vi "stop.vi"(8 "error in (no error)":errorcluster, 11 "control references in":T1) -> (0 "error out":errorcluster, 3 "control references out":T1)   [LabVIEW 2010]
uses:
  type_definitions/clusters/controls_refs.ctl
  common/classes/GenericToplevelComponent/GenericToplevelComponent/GenericToplevelComponent.lvclass
  type_definitions/enumerations/main_control_types.ctl
  components/ImagingMode/GenericImagingMode/GenericImagingMode/GenericImagingMode.lvclass
  components/ExperimentController/GenericExperimentController/GenericExperimentController/GenericExperimentController.lvclass
  global_variables.vi
  common/classes/GenericComponent/GenericComponent/class_data.vi
  common/classes/GenericComponent/GenericComponent/GenericComponent.lvclass
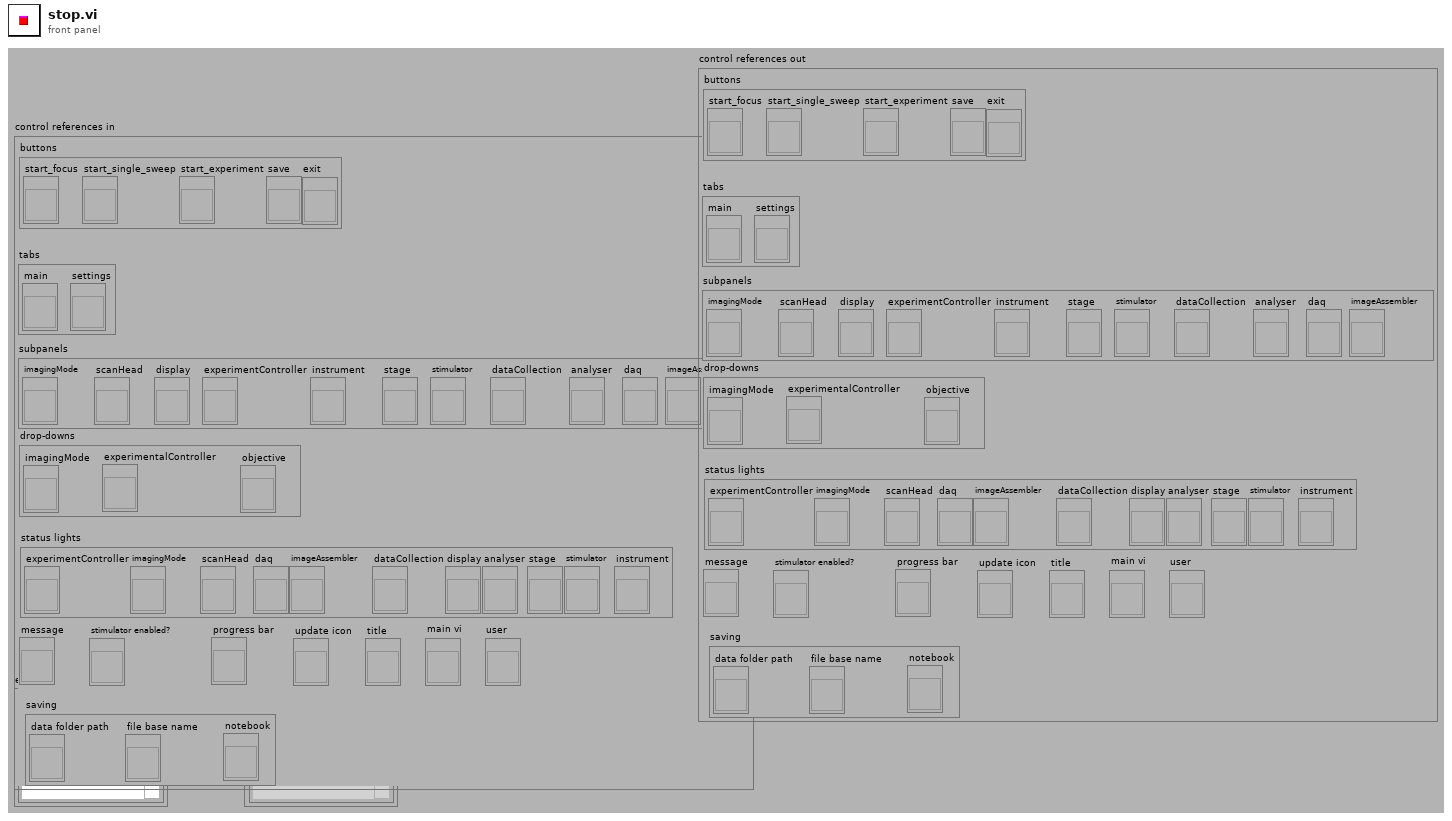
[diagram p1: front panel]
types:
  T1 = typedef "controls_refs.ctl" = cluster{"buttons":cluster{"start_focus":refnum<vi>, "start_single_sweep":refnum<vi>, "start_experiment":refnum<vi>, "save":refnum<vi>, "exit":refnum<vi>}, "tabs":cluster{"main":refnum<vi>, "settings":refnum<vi>}, "subpanels":cluster{"imagingMode":refnum<vi>, "scanHead":refnum<vi>, "display":refnum<vi>, "experimentController":refnum<vi>, "instrument":refnum<vi>, "stage":refnum<vi>, "stimulator":refnum<vi>, "dataCollection":refnum<vi>, "analyser":refnum<vi>, "daq":refnum<vi>, "imageAssembler":refnum<vi>}, "drop-downs":cluster{"imagingMode":refnum<vi>, "experimentalController":refnum<vi>, "objective":refnum<vi>}, "status lights":cluster{"experimentController":refnum<vi>, "imagingMode":refnum<vi>, "scanHead":refnum<vi>, "daq":refnum<vi>, "imageAssembler":refnum<vi>, "dataCollection":refnum<vi>, "display":refnum<vi>, "analyser":refnum<vi>, "stage":refnum<vi>, "stimulator":refnum<vi>, "instrument":refnum<vi>}, "message":refnum<vi>, "stimulator enabled?":refnum<vi>, "saving":cluster{"data folder path":refnum<vi>, "file base name":refnum<vi>, "notebook":refnum<vi>}, "progress bar":refnum<vi>, "update icon":refnum<vi>, "title":refnum<vi>, "main vi":refnum<vi>, "user":refnum<vi>}
  T2 = enum8{"Enabled", "Disabled", "Disabled and Grayed Out"}
  T3 = typedef "main_control_types.ctl" = enum16{"scan start button", "experimentController subpanel", "imagingMode subpanel", "scanHead subpanel", "dataCollection subpanel", "display subpanel", "analyser subpanel", "stimulator subpanel", "imagingMode drop-down", "experimentController drop-down", "objective drop-down", "exit button"}
  T4 = typedef "GenericToplevelComponent.lvclass/common_trigger_enum.ctl" = enum16{"NULL", "initialise", "terminate", "fetch command", "fetch data", "attach observer", "register as observer", "detach observer", "acknowledge", "start", "stop", "sweep started", "sweep finished", "experiment started", "experiment stopped"}
  T5 = typedef "run_mode_enum.ctl" = enum16{"focus mode", "single sweep mode", "experiment mode"}
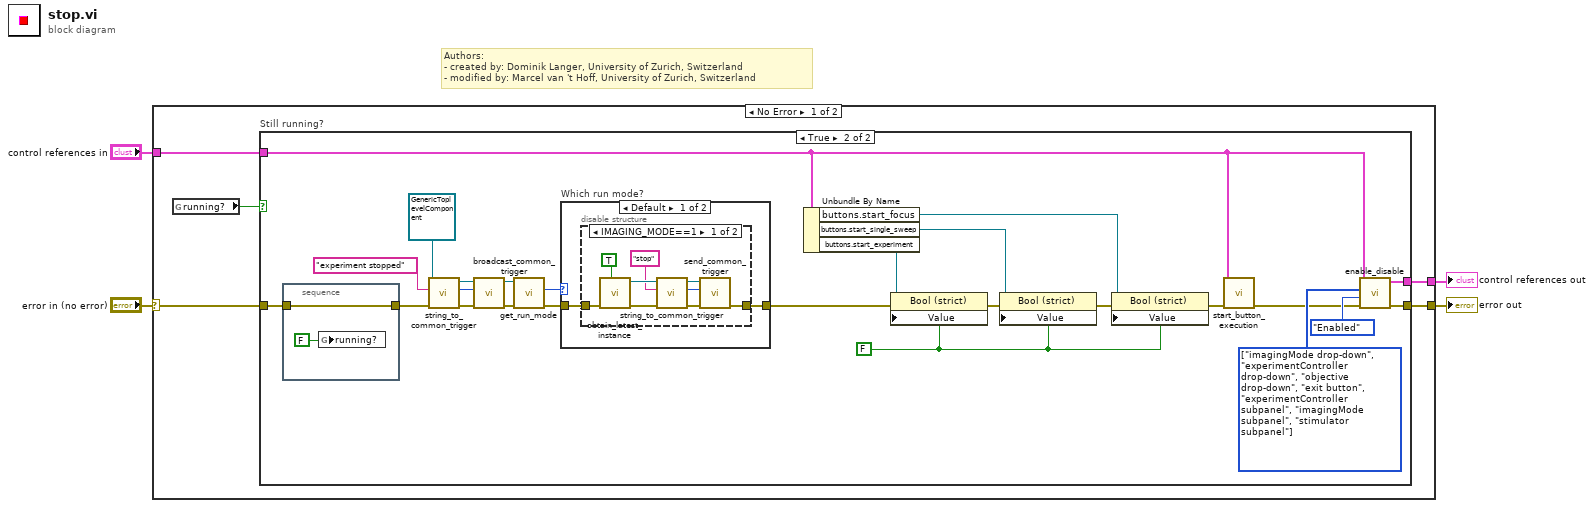
[diagram p0: block diagram]
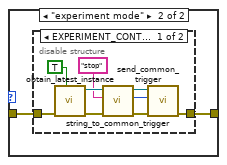
[diagram p4: hidden frame]
diagram:
  # "Authors: \n- created by: Dominik Langer, University of Zurich, Switzerland\n- modified by: Marcel van 't Hoff, University of Zurich, Switzerland"
  n1 = case shown="No Error" "error in (no error)" {
    selector: "error in (no error)" -> [w9 w63]
    tunnel: [w6 w63] -> w3
    tunnel: "control references in" -> [w8 w62]
    tunnel: [w7 w62] -> w1
    frame No Error {
      n2 = global read "global_variables.vi" "running?"() -> (w5:bool)
      n3 = case "Still running?" shown="True" w5 {
        tunnel: w9 -> [w11 w34]
        tunnel: w8 -> [w10 w13]
        tunnel: [w10 w32] -> w7
        tunnel: [w11 w31] -> w6
        frame False {
        }
        frame True {
          w18 = FALSE
          w33 = T3[] [enum."imagingMode drop-down", enum."experimentController drop-down", enum."objective drop-down", enum."exit button", enum."experimentController subpanel", enum."imagingMode subpanel", enum."stimulator subpanel"] items=["scan start button", "experimentController subpanel", "imagingMode subpanel", "scanHead subpanel", "dataCollection subpanel", "display subpanel", "analyser subpanel", "stimulator subpanel", "imagingMode drop-down", "experimentController drop-down", "objective drop-down", "exit button"] ("controls")
          n4 = stacked-sequence {
            tunnel: w34 -> [w38]
            tunnel: [w38] -> w25
            frame #0 {
              n5 = global write "global_variables.vi" "running?"(FALSE) -> ()
            }
          }
          n6 = call-dynamic "string_to_common_trigger.vi"("error in (no error)"=w25, "trigger string"="experiment stopped", "GenericToplevelComponent in"=refnum<class "GenericToplevelComponent.lvclass"> refnum ("GenericToplevelComponent.lvclass")) -> ("error out"=w24:errorcluster, "trigger"=w23:T4, "GenericToplevelComponent out"=w26:refnum<class "GenericToplevelComponent.lvclass">)  [unwired: 6 in]
          n7 = call-dynamic "broadcast_common_trigger.vi"("error in (no error)"=w24, "trigger"=w23, "GenericToplevelComponent in"=w26) -> ("error out"=w29:errorcluster, "GenericToplevelComponent out"=w28:refnum<class "GenericToplevelComponent.lvclass">)  [unwired: 7 in]
          n8 = call "get_run_mode.vi"("error in (no error)"=w29, "GenericPlugin in"=w28) -> ("error out"=w36:errorcluster, "run mode"=w35:T5)  [unwired: 5 in, 3 out]
          n9 = case "Which run mode?" shown="Default" w35 {
            tunnel: [w40 w51] -> w12
            tunnel: w36 -> [w39 w52]
            frame Default {
              n10 = disable-structure shown="IMAGING_MODE==1" {
                disable-tunnel: w39 -> [w49 w50]
                disable-tunnel: [w48 w50] -> w40
                frame condition #0 (active) {
                  n11 = call "obtain_latest_instance.vi"("quick, but maybe outdated?"=TRUE, "error in (no error)"=w49) -> ("error out"=w42:errorcluster, "GenericScanMode out"=w46:refnum<class "GenericImagingMode.lvclass">)  [unwired: 8 out]
                  n12 = call-dynamic "string_to_common_trigger.vi"("error in (no error)"=w42, "trigger string"="stop", "GenericToplevelComponent in"=w46) -> ("error out"=w43:errorcluster, "trigger"=w44:T4, "GenericToplevelComponent out"=w45:refnum<class "GenericImagingMode.lvclass">)  [unwired: 6 in]
                  n13 = call-dynamic "send_common_trigger.vi"("error in (no error)"=w43, "trigger"=w44, "GenericToplevelComponent in"=w45) -> ("error out"=w48:errorcluster)  [unwired: 6 in, 2 out]
                }
                frame condition #1 {
                }
              }
            }
            frame "experiment mode" {
              n14 = disable-structure shown="EXPERIMENT_CONTROLLER==1" {
                disable-tunnel: w52 -> [w60 _]
                disable-tunnel: [w59 _] -> w51
                frame condition #0 (active) {
                  n15 = call "obtain_latest_instance.vi"("quick, but maybe outdated?"=TRUE, "error in (no error)"=w60) -> ("error out"=w56:errorcluster, "GenericExperimentController out"=w57:refnum<class "GenericExperimentController.lvclass">)  [unwired: 8 in]
                  n16 = call-dynamic "string_to_common_trigger.vi"("error in (no error)"=w56, "trigger string"="stop", "GenericToplevelComponent in"=w57) -> ("error out"=w55:errorcluster, "trigger"=w54:T4, "GenericToplevelComponent out"=w58:refnum<class "GenericExperimentController.lvclass">)  [unwired: 6 in]
                  n17 = call-dynamic "send_common_trigger.vi"("error in (no error)"=w55, "trigger"=w54, "GenericToplevelComponent in"=w58) -> ("error out"=w59:errorcluster)  [unwired: 6 in, 2 out]
                }
                frame condition #1 {
                }
              }
            }
          }
          n18 = Unbundle By Name(w13) -> ("buttons.start_focus"=w21:refnum<vi>, "buttons.start_single_sweep"=w19:refnum<vi>, "buttons.start_experiment"=w20:refnum<vi>)
          n19 = property class="Bool (strict)"(reference=w20, error in=w12, "Value"=w18) -> (error out=w16:errorcluster)  [unwired: 1 out]
          n20 = property class="Bool (strict)"(reference=w19, error in=w16, "Value"=w18) -> (error out=w15:errorcluster)  [unwired: 1 out]
          n21 = property class="Bool (strict)"(reference=w21, error in=w15, "Value"=w18) -> (error out=w14:errorcluster)  [unwired: 1 out]
          n22 = call "start_button_execution.vi"("error in (no error)"=w14, "control references"=w13) -> ("error out"=w17:errorcluster)  [unwired: 7 in, 2 out]
          n23 = call "enable_disable.vi"("error in (no error)"=w17, "state"=T2."Enabled" ("Disabled"), "controls"=w33, "control references in"=w13) -> ("error out"=w31:errorcluster, "control references out"=w32:T1)  [unwired: 6 in]
        }
      }
    }
    frame Error {
    }
  }
  "error out" <- w3
  "control references out" <- w1
